vi "Test.vi"() -> ()   [LabVIEW 2025]
panel:
  out "B":fxp<+/-,64,32>[](array[numeric])
  in  "A":fxp<+/-,64,32>[](array[numeric])
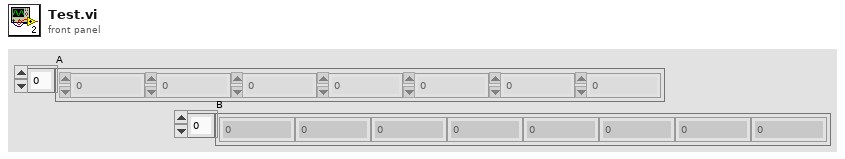
[diagram p1: front panel]
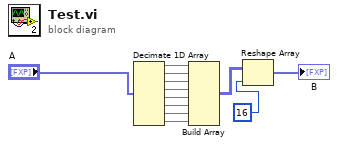
[diagram p0: block diagram]
diagram:
  n1 = Decimate 1D Array("A") -> (w12:fxp<+/-,64,32>[], w11:fxp<+/-,64,32>[], w10:fxp<+/-,64,32>[], w9:fxp<+/-,64,32>[], w8:fxp<+/-,64,32>[], w7:fxp<+/-,64,32>[], w6:fxp<+/-,64,32>[], w5:fxp<+/-,64,32>[])
  n2 = Build Array(w12, w11, w10, w9, w8, w7, w6, w5) -> (w4:fxp<+/-,64,32>[][])
  n3 = Reshape Array(w4, 16 ("dimension size")) -> (→"B":fxp<+/-,64,32>[])
